vi "XYGraph.CreateErrorBars.vi"(0 "xTemp":dbl, 5 "yTemp":dbl, 7 "errorTemp":dbl) -> (4 "error bar plot":cluster{dbl[], dbl[]} {"?" format="%.2f"; "?" format="%.2f"})   [LabVIEW 2012]
doc: "Creates a error bar plot\n\nwww.sciware.com.au"
panel:
  in  "error":dbl[](array[numeric]) format="%.2f"
  in  "Y":dbl[](array[numeric]) format="%.2f"
  in  "X":dbl[](array[numeric]) format="%.2f"
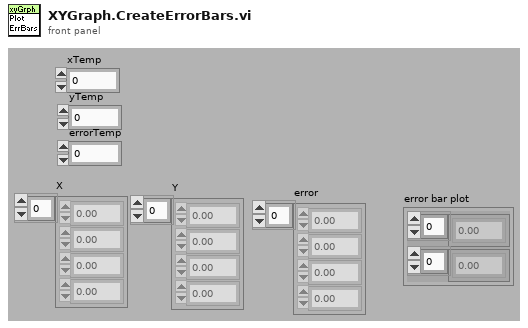
[diagram p1: front panel]
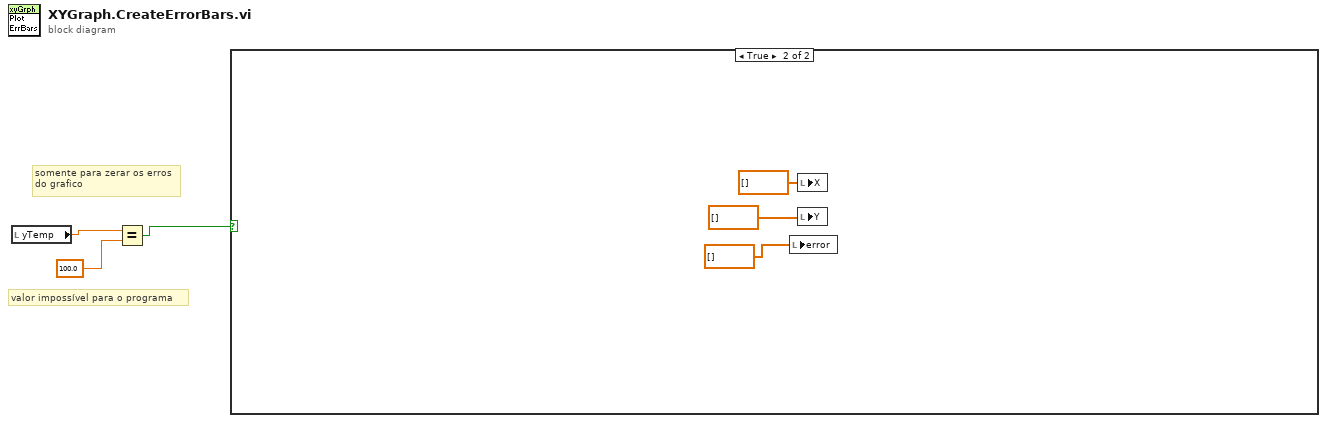
[diagram p0: block diagram]
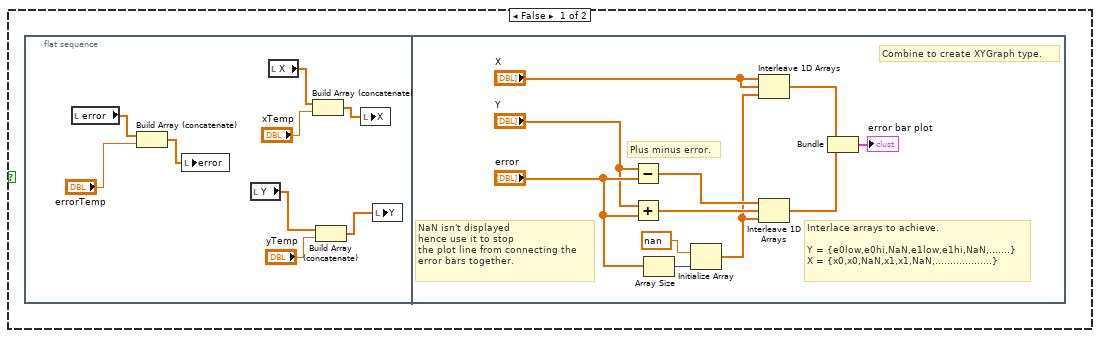
[diagram p2: hidden frame]
diagram:
  # "valor impossível para o programa"
  # "somente para zerar os erros\ndo grafico"
  n1 = local read "yTemp"() -> (w3:dbl)
  n2 = Equal?(x=w3, y=100.0) -> (x = y?=w1:bool)
  n3 = case shown="True" w1 {
    frame False {
      n4 = flat-sequence {
        frame #0 {
          n5 = local read "error"() -> (w6:dbl[])
          n6 = Build Array (concatenate)(w6, "errorTemp") -> (w4:dbl[])
          n7 = local write "error"(w4) -> ()
          n8 = local read "Y"() -> (w9:dbl[])
          n9 = local read "X"() -> (w12:dbl[])
          n10 = Build Array (concatenate)(w12, "xTemp") -> (w10:dbl[])
          n11 = Build Array (concatenate)(w9, "yTemp") -> (w7:dbl[])
          n12 = local write "X"(w10) -> ()
          n13 = local write "Y"(w7) -> ()
        }
        frame #1 {
          # "Interlace arrays to achieve.\n\nY = {e0low,e0hi,NaN,e1low,e1hi,NaN,.......}\nX = {x0,x0,NaN,x1,x1,NaN,...................}"
          # "NaN isn't displayed\nhence use it to stop\nthe plot line from connecting the\nerror bars together."
          # "Combine to create XYGraph type."
          # "Plus minus error."
          n14 = Subtract(x="Y", y="error") -> (x-y=w23:dbl[])
          n15 = Add(x="Y", y="error") -> (x+y=w22:dbl[])
          n16 = Array Size(array="error") -> (size(s)=w21:i32)
          n17 = Initialize Array(nan ("element"), w21) -> (w18:dbl[])
          n18 = Interleave 1D Arrays("X", "X", w18) -> (w15:dbl[])
          n19 = Interleave 1D Arrays(w23, w22, w18) -> (w14:dbl[])
          n20 = Bundle(w15, w14) -> (→"error bar plot":cluster{dbl[], dbl[]})  [unwired: 1 in]
        }
      }
    }
    frame True {
      n21 = local write "error"(dbl[] [] ("X")) -> ()
      n22 = local write "X"(dbl[] [] ("X")) -> ()
      n23 = local write "Y"(dbl[] [] ("X")) -> ()
    }
  }
